vi "Queue Stack Maze Solver.vi"() -> ()   [LabVIEW 2016]
doc: "Implements a maze solver using a queue stack. Specifically, this VI demonstrates the Enqueue Element At Opposite End function to keep the solved portion of the maze within the queue."
uses:
  Support Files/Queue Stack Maze - Square Color.ctl
  Support Files/Queue Stack Maze - Position.ctl
  Support Files/Queue Stack Maze - Direction.ctl
  Support Files/Queue Stack Maze - Square Meaning.ctl
panel:
  out "Maze":T1[][](array[typedef])
  # "Overview: Demonstrates the use of the Queue functions to implement a stack-based maze solver.\nInstructions:\nRun the VI."
  # "Color Legend:\n\nBlack - Wall\nGreen - Unexplored path\nBlue - Explored path (not yet rejected)\nRed - Rejected path\nPurple - Ending space\nYellow - Solved path (generated when maze is completely solved)"
  # "As the solver runs, it displays the state of each square in the maze. As different paths are explored, they will turn blue. If a path is rejected, it will turn red, and the solver will backtrack to find another unexplored path."
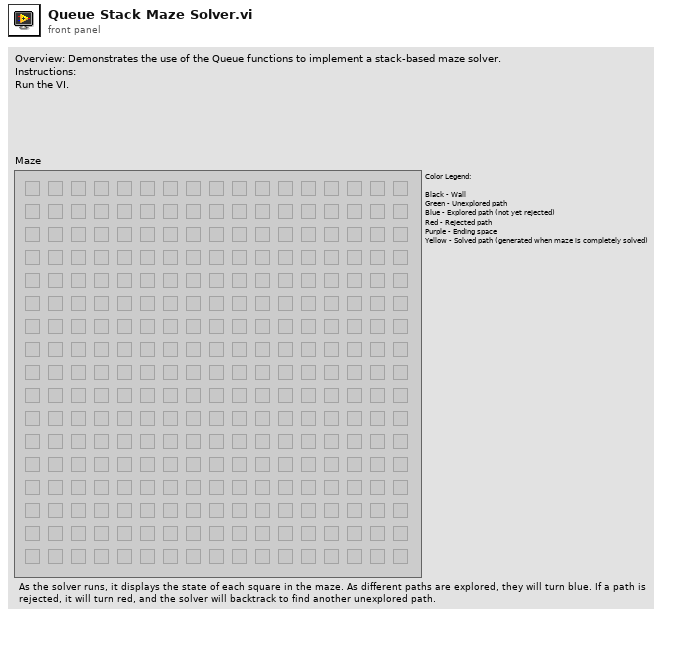
[diagram p1: front panel]
types:
  T1 = typedef "Queue Stack Maze - Square Color.ctl" = u16
  T2 = typedef "Queue Stack Maze - Square Meaning.ctl" = enum16{"Open", "Wall", "Path", "Rejected", "Ending", "Checking North", "Checking South", "Checking East", "Checking West"}
  T3 = typedef "Queue Stack Maze - Position.ctl" = cluster{"Row":i32, "Column":i32, "Went":T4}
  T4 = typedef "Queue Stack Maze - Direction.ctl" = enum16{"North", "South", "East", "West"}
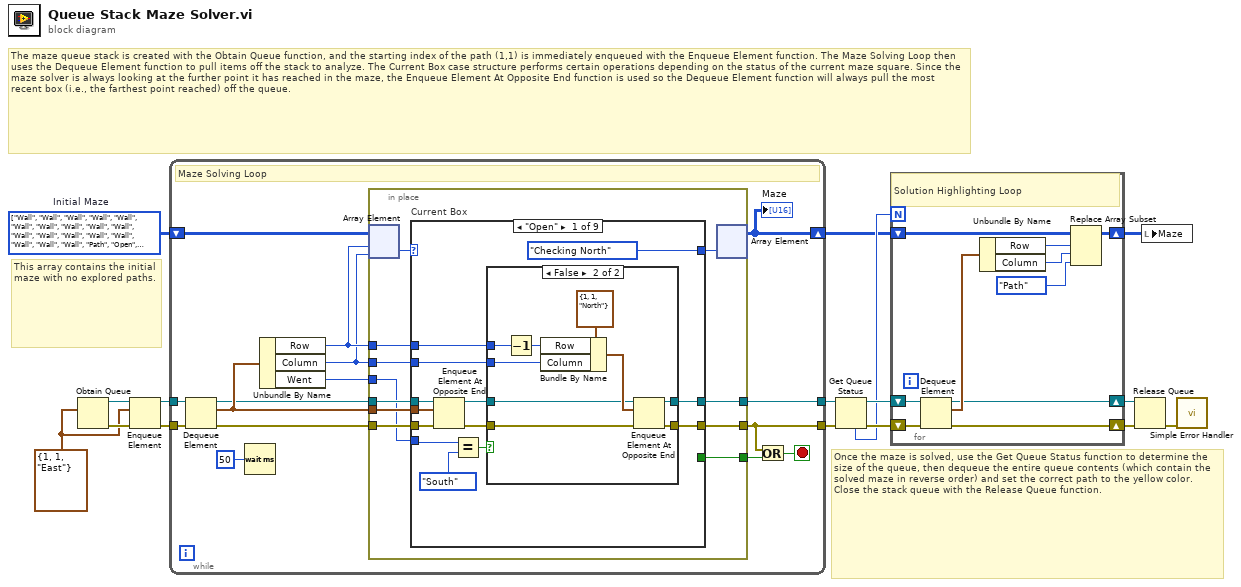
[diagram p0: block diagram]
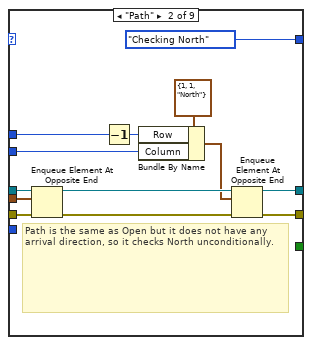
[diagram p3: hidden frame]
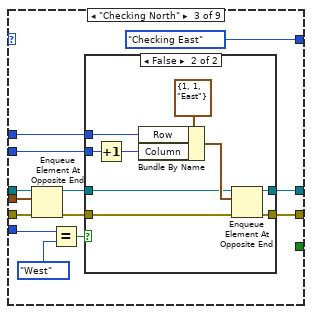
[diagram p4: hidden frame]
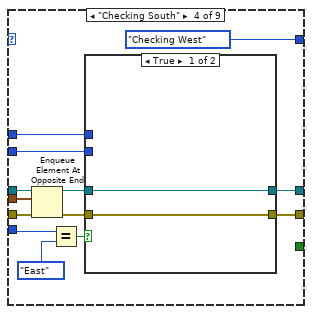
[diagram p6: hidden frame]
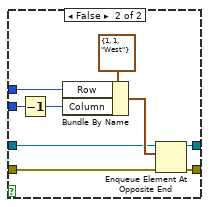
[diagram p7: hidden frame]
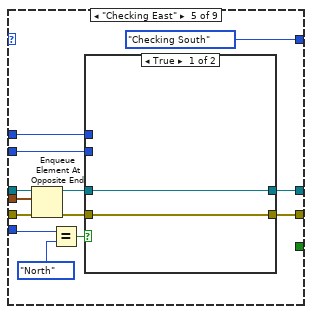
[diagram p8: hidden frame]
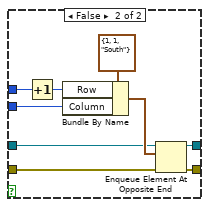
[diagram p9: hidden frame]
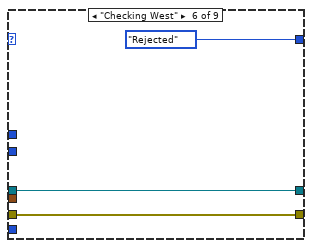
[diagram p10: hidden frame]
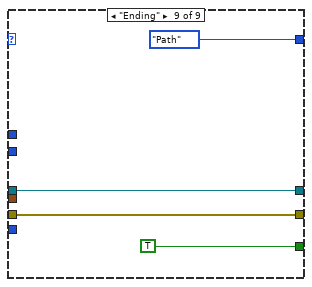
[diagram p13: hidden frame]
diagram:
  w11 = T2[][] [[enum."Wall", enum."Wall", enum."Wall", enum."Wall", enum."Wall", enum."Wall", enum."Wall", enum."Wall", enum."Wall", enum."Wall", enum."Wall", enum."Wall", enum."Wall", enum."Wall", enum."Wall", enum."Wall", enum."Wall"], [enum."Wall", enum."Path", enum."Open", enum."Open", enum."Wall", enum."Open", enum."Open", enum."Open", enum."Open", enum."Open", enum."Wall", enum."Open", enum."Open", enum."Open", enum."Open", enum."Open", enum."Wall"], [enum."Wall", enum."Wall", enum."Wall", enum."Open", enum."Open", enum."Open", enum."Wall", enum."Open", enum."Wall", enum."Open", enum."Wall", enum."Open", enum."Wall", enum."Wall", enum."Wall", enum."Wall", enum."Wall"], [enum."Wall", enum."Open", enum."Open", enum."Open", enum."Wall", enum."Open", enum."Wall", enum."Wall", enum."Open", enum."Open", enum."Open", enum."Open", enum."Open", enum."Open", enum."Open", enum."Open", enum."Wall"], [enum."Wall", enum."Open", enum."Wall", enum."Wall", enum."Wall", enum."Open", enum."Open", enum."Open", enum."Wall", enum."Open", enum."Wall", enum."Wall", enum."Open", enum."Wall", enum."Wall", enum."Wall", enum."Wall"], [enum."Wall", enum."Open", enum."Open", enum."Open", enum."Wall", enum."Wall", enum."Wall", enum."Open", enum."Wall", enum."Open", enum."Open", enum."Open", enum."Wall", enum."Open", enum."Open", enum."Open", enum."Wall"], [enum."Wall", enum."Open", enum."Wall", enum."Wall", enum."Open", enum."Open", enum."Open", enum."Open", enum."Wall", enum."Wall", enum."Wall", enum."Open", enum."Wall", enum."Open", enum."Wall", enum."Open", enum."Wall"], [enum."Wall", enum."Open", enum."Open", enum."Open", enum."Wall", enum."Open", enum."Wall", enum."Wall", enum."Wall", enum."Open", enum."Open", enum."Wall", enum."Open", enum."Wall", enum."Wall", enum."Open", enum."Wall"], [enum."Wall", enum."Open", enum."Wall", enum."Open", enum."Wall", enum."Open", enum."Wall", enum."Open", enum."Wall", enum."Open", enum."Wall", enum."Open", enum."Open", enum."Open", enum."Open", enum."Open", enum."Wall"], [enum."Wall", enum."Open", enum."Wall", enum."Open", enum."Wall", enum."Open", enum."Wall", enum."Open", enum."Wall", enum."Open", enum."Wall", enum."Open", enum."Wall", enum."Open", enum."Wall", enum."Open", enum."Wall"], [enum."Wall", enum."Wall", enum."Wall", enum."Wall", enum."Wall", enum."Open", enum."Wall", enum."Open", enum."Wall", enum."Open", enum."Open", enum."Open", enum."Wall", enum."Open", enum."Open", enum."Wall", enum."Wall"], [enum."Wall", enum."Open", enum."Open", enum."Open", enum."Open", enum."Open", enum."Wall", enum."Open", enum."Open", enum."Wall", enum."Wall", enum."Open", enum."Wall", enum."Wall", enum."Open", enum."Open", enum."Wall"], [enum."Wall", enum."Open", enum."Wall", enum."Wall", enum."Open", enum."Wall", enum."Wall", enum."Open", enum."Open", enum."Open", enum."Wall", enum."Open", enum."Open", enum."Open", enum."Wall", enum."Open", enum."Wall"], [enum."Wall", enum."Open", enum."Wall", enum."Open", enum."Open", enum."Open", enum."Wall", enum."Open", enum."Wall", enum."Open", enum."Open", enum."Open", enum."Wall", enum."Open", enum."Wall", enum."Open", enum."Wall"], [enum."Wall", enum."Open", enum."Wall", enum."Open", enum."Wall", enum."Open", enum."Wall", enum."Open", enum."Wall", enum."Wall", enum."Wall", enum."Wall", enum."Wall", enum."Wall", enum."Open", enum."Open", enum."Wall"], [enum."Wall", enum."Open", enum."Open", enum."Wall", enum."Open", enum."Open", enum."Open", enum."Open", enum."Open", enum."Open", enum."Open", enum."Open", enum."Open", enum."Open", enum."Wall", enum."Ending", enum."Wall"], [enum."Wall", enum."Wall", enum."Wall", enum."Wall", enum."Wall", enum."Wall", enum."Wall", enum."Wall", enum."Wall", enum."Wall", enum."Wall", enum."Wall", enum."Wall", enum."Wall", enum."Wall", enum."Wall", enum."Wall"]] items=["Open", "Wall", "Path", "Rejected", "Ending", "Checking North", "Checking South", "Checking East", "Checking West"]  # Initial Maze
  w14 = T3 {"Row"=1, "Column"=1, "Went"=enum."East"}
  # "The maze queue stack is created with the Obtain Queue function, and the starting index of the path (1,1) is immediately enqueued with the Enqueue Element function. The Maze Solving Loop then uses the Dequeue Element function to pull items off the stack to analyze. The Current Box case structure performs certain operations depending on the status of the current maze square. Since the maze solver is always looking at the further point it has reached in the maze, the Enqueue Element At Opposite End function is used so the Dequeue Element function will always pull the most recent box (i.e., the farthest point reached) off the queue."
  # "This array contains the initial maze with no explored paths."
  # "Once the maze is solved, use the Get Queue Status function to determine the size of the queue, then dequeue the entire queue contents (which contain the solved maze in reverse order) and set the correct path to the yellow color. Close the stack queue with the Release Queue function."
  n1 = Obtain Queue(element data type=w14) -> (queue out=w16:refnum<queue>, error out=w15:errorcluster)  [unwired: 3 in, 2 out]
  n2 = Enqueue Element(queue=w16, element=w14, error in (no error)=w15) -> (queue out=w12:refnum<queue>, error out=w13:errorcluster)  [unwired: 2 out]
  n3 = while "While Loop - Find the path" {
    shift-right: [w18] -> w2
    shift-left: w11 -> [w21]
    tunnel: w12 -> [w30]
    tunnel: w13 -> [w31]
    tunnel: [w22] -> w6
    tunnel: [w17] -> w7
    stop <- w23 stop-if-true
    # "Maze Solving Loop"
    n4 = Dequeue Element(queue=w30, error in (no error)=w31) -> (queue out=w27:refnum<queue>, element=w28:T3, error out=w29:errorcluster)  [unwired: 1 in, 1 out]
    n5 = Wait (ms)(milliseconds to wait=u32 50) -> ()  [unwired: 1 out]
    n6 = Unbundle By Name(w28) -> ("Row"=w20:i32, "Column"=w19:i32, "Went"=w25:T4)
    n7 = in-place {
      in-place-border: w29 -> [w42]
      in-place-border: w28 -> [w41]
      in-place-border: w27 -> [w40]
      in-place-border: w25 -> [w39]
      in-place-border: w20 -> [w38]
      in-place-border: w19 -> [w37]
      in-place-border: [w36] -> w24
      in-place-border: [w35] -> w22
      in-place-border: [w32] -> w17
      n8 = in-place-array #1(w21, w20, w19) -> (w34:T2)
      n9 = case "Current Box" shown="\"Open\"" w34 {
        selector: w34 -> [_ _ _ _ _ _ w157 w160 _]
        tunnel: [_ _ _ _ _ _ _ _ TRUE] -> w36
        tunnel: [Queue_Stack_Maze_-_Square_Meaning."Checking North" ("Enum") Queue_Stack_Maze_-_Square_Meaning."Checking North" ("Enum") Queue_Stack_Maze_-_Square_Meaning."Checking East" ("Enum") Queue_Stack_Maze_-_Square_Meaning."Checking West" ("Enum") Queue_Stack_Maze_-_Square_Meaning."Checking South" ("Enum") Queue_Stack_Maze_-_Square_Meaning."Rejected" ("Enum") w157 w160 Queue_Stack_Maze_-_Square_Meaning."Path" ("Enum")] -> w33
        tunnel: w40 -> [w53 w77 w90 w114 w138 w152 w155 w158 w161]
        tunnel: w38 -> [w49 w73 w86 w110 w134 _ _ _ _]
        tunnel: w37 -> [w54 w78 w91 w115 w139 _ _ _ _]
        tunnel: w42 -> [w51 w75 w88 w112 w136 w153 w156 w159 w162]
        tunnel: w41 -> [w48 w72 w85 w109 w133 _ _ _ _]
        tunnel: w39 -> [w46 _ w83 w107 w131 _ _ _ _]
        tunnel: [w44 w68 w81 w105 w129 w153 w156 w159 w162] -> w35
        tunnel: [w43 w67 w80 w104 w128 w152 w155 w158 w161] -> w32
        frame "Open" {
          n10 = Enqueue Element At Opposite End(queue=w53, element=w48, error in (no error)=w51) -> (queue out=w52:refnum<queue>, error out=w50:errorcluster)  [unwired: 2 out]
          n11 = Equal?(x=w46, y=Queue_Stack_Maze_-_Direction."South" ("Went")) -> (x = y?=w47:bool)
          n12 = case shown="False" w47 {
            tunnel: w54 -> [_ w61]
            tunnel: w52 -> [w56 w65]
            tunnel: w50 -> [w57 w64]
            tunnel: w49 -> [_ w63]
            tunnel: [w57 w59] -> w44
            tunnel: [w56 w58] -> w43
            frame True {
            }
            frame False {
              n13 = Decrement(x=w63) -> (x-1=w60:i32)
              n14 = Bundle By Name(cluster=T3 {"Row"=1, "Column"=1, "Went"=enum."North"}, "Row"=w60, "Column"=w61) -> (w66:T3)
              n15 = Enqueue Element At Opposite End(queue=w65, element=w66, error in (no error)=w64) -> (queue out=w58:refnum<queue>, error out=w59:errorcluster)  [unwired: 2 out]
            }
          }
        }
        frame "Path" {
          # "Path is the same as Open but it does not have any arrival direction, so it checks North unconditionally."
          n16 = Enqueue Element At Opposite End(queue=w77, element=w72, error in (no error)=w75) -> (queue out=w76:refnum<queue>, error out=w74:errorcluster)  [unwired: 2 out]
          n17 = Decrement(x=w73) -> (x-1=w69:i32)
          n18 = Bundle By Name(cluster=T3 {"Row"=1, "Column"=1, "Went"=enum."North"}, "Row"=w69, "Column"=w78) -> (w71:T3)
          n19 = Enqueue Element At Opposite End(queue=w76, element=w71, error in (no error)=w74) -> (queue out=w67:refnum<queue>, error out=w68:errorcluster)  [unwired: 2 out]
        }
        frame "Checking North" {
          n20 = Enqueue Element At Opposite End(queue=w90, element=w85, error in (no error)=w88) -> (queue out=w89:refnum<queue>, error out=w87:errorcluster)  [unwired: 2 out]
          n21 = Equal?(x=w83, y=Queue_Stack_Maze_-_Direction."West" ("Went")) -> (x = y?=w84:bool)
          n22 = case shown="False" w84 {
            tunnel: w91 -> [_ w99]
            tunnel: w89 -> [w93 w102]
            tunnel: w87 -> [w94 w101]
            tunnel: w86 -> [_ w98]
            tunnel: [w94 w96] -> w81
            tunnel: [w93 w95] -> w80
            frame True {
            }
            frame False {
              n23 = Increment(x=w99) -> (x+1=w97:i32)
              n24 = Bundle By Name(cluster=T3 {"Row"=1, "Column"=1, "Went"=enum."East"}, "Row"=w98, "Column"=w97) -> (w103:T3)
              n25 = Enqueue Element At Opposite End(queue=w102, element=w103, error in (no error)=w101) -> (queue out=w95:refnum<queue>, error out=w96:errorcluster)  [unwired: 2 out]
            }
          }
        }
        frame "Checking South" {
          n26 = Enqueue Element At Opposite End(queue=w114, element=w109, error in (no error)=w112) -> (queue out=w113:refnum<queue>, error out=w111:errorcluster)  [unwired: 2 out]
          n27 = Equal?(x=w107, y=Queue_Stack_Maze_-_Direction."East" ("Went")) -> (x = y?=w108:bool)
          n28 = case shown="True" w108 {
            tunnel: w115 -> [_ w126]
            tunnel: w113 -> [w117 w125]
            tunnel: w111 -> [w118 w124]
            tunnel: w110 -> [_ w123]
            tunnel: [w118 w120] -> w105
            tunnel: [w117 w119] -> w104
            frame True {
            }
            frame False {
              n29 = Decrement(x=w126) -> (x-1=w122:i32)
              n30 = Bundle By Name(cluster=T3 {"Row"=1, "Column"=1, "Went"=enum."West"}, "Row"=w123, "Column"=w122) -> (w127:T3)
              n31 = Enqueue Element At Opposite End(queue=w125, element=w127, error in (no error)=w124) -> (queue out=w119:refnum<queue>, error out=w120:errorcluster)  [unwired: 2 out]
            }
          }
        }
        frame "Checking East" {
          n32 = Enqueue Element At Opposite End(queue=w138, element=w133, error in (no error)=w136) -> (queue out=w137:refnum<queue>, error out=w135:errorcluster)  [unwired: 2 out]
          n33 = Equal?(x=w131, y=Queue_Stack_Maze_-_Direction."North" ("Went")) -> (x = y?=w132:bool)
          n34 = case shown="True" w132 {
            tunnel: w139 -> [_ w146]
            tunnel: w137 -> [w141 w150]
            tunnel: w135 -> [w142 w149]
            tunnel: w134 -> [_ w148]
            tunnel: [w142 w144] -> w129
            tunnel: [w141 w143] -> w128
            frame True {
            }
            frame False {
              n35 = Increment(x=w148) -> (x+1=w145:i32)
              n36 = Bundle By Name(cluster=T3 {"Row"=1, "Column"=1, "Went"=enum."South"}, "Row"=w145, "Column"=w146) -> (w151:T3)
              n37 = Enqueue Element At Opposite End(queue=w150, element=w151, error in (no error)=w149) -> (queue out=w143:refnum<queue>, error out=w144:errorcluster)  [unwired: 2 out]
            }
          }
        }
        frame "Checking West" {
        }
        frame "Wall" {
        }
        frame "Rejected" {
          # "Do nothing when a Rejected square is encountered. The next most recent square on the current path will be checked on the next iteration."
        }
        frame "Ending" {
        }
      }
      n38 = in-place-array #1(w33) -> (w18:T2[][])  [unwired: 2 out]
    }
    "Maze" <- w18
    n39 = Or(x=w22, y=w24) -> (x .or. y?=w23:bool)
  }
  n40 = Get Queue Status(queue=w7, error in (no error)=w6) -> (queue out=w10:refnum<queue>, error out=w9:errorcluster, # elements in queue=w8:i32)  [unwired: 6 out]
  n41 = for {
    N: w8 -> [_]
    shift-right: [w171] -> w1
    shift-left: w2 -> [w172]
    shift-right: [w166] -> w4
    shift-left: w9 -> [w173]
    shift-right: [w165] -> w3
    shift-left: w10 -> [w174]
    # "Solution Highlighting Loop"
    n42 = Dequeue Element(queue=w174, error in (no error)=w173) -> (queue out=w165:refnum<queue>, element=w170:T3, error out=w166:errorcluster)  [unwired: 2 out]
    n43 = Unbundle By Name(w170) -> ("Row"=w169:i32, "Column"=w168:i32)
    n44 = Replace Array Subset(array=w172, new element=Queue_Stack_Maze_-_Square_Meaning."Path" ("Enum"), index (row)=w169, index (col)=w168) -> (w171:T2[][])
  }
  n45 = Release Queue(queue=w3, error in (no error)=w4) -> (error out=w5:errorcluster)  [unwired: 1 in, 2 out]
  n46 = local write "Maze"(w1) -> ()
  n47 = call <vilib>:"Simple Error Handler.vi"("error in (no error)"=w5) -> ()  [unwired: 4 in, 5 out]
